vi "Save data to file polymorphic.vi"   [LabVIEW 2018]
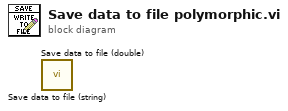
[diagram p0: block diagram]
diagram:
  n1 = call "Save data to file (string).vi"() -> ()  [unwired: 12 in]
  n2 = call "Save data to file (double).vi"() -> ()  [unwired: 12 in]
